vi "sg Get Serial Number.vi"(8 "error in (no error)":errorcluster, 10 "serialNumber":i32, 11 "device":i32) -> (0 "error out":errorcluster, 2 "serialNumber out":i32, 3 "function return":u32(ring))   [LabVIEW 2014, in "VSG25A.lvlib"]
doc: "SG_API sgStatus sgGetSerialNumber(int device, int *serialNumber);"
uses:
  VSG25A.lvlib
  sg_api.dll
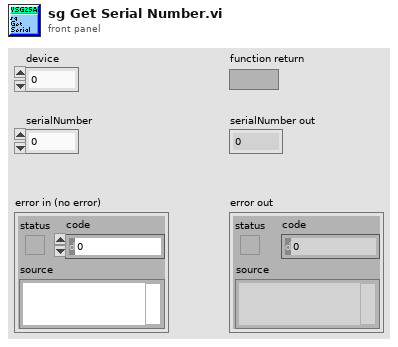
[diagram p1: front panel]
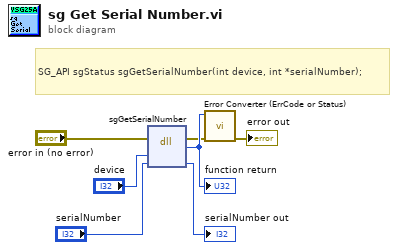
[diagram p0: block diagram]
diagram:
  # "SG_API sgStatus sgGetSerialNumber(int device, int *serialNumber);"
  n1 = dll-call lib="C:/Users/M_LAPTOP/Desktop/Labview/practice/VSG25A/sg_lib/sg_api.*" fn="sgGetSerialNumber"(error in="error in (no error)", "device"="device", "serialNumber"="serialNumber") -> (error out=w2:errorcluster, w7:u32, "serialNumber"=→"serialNumber out":i32)  [unwired: 3 in, 1 out]
  "function return" <- w7
  n2 = call "Error Converter (ErrCode or Status).vi"("error in (no error)"=w2, "error code"=w7) -> ("error out"=→"error out":errorcluster)  [unwired: 9 in]
